vi "Channel by Index.vi"(8 "error in (no error)":errorcluster, 10 "Index":i32, 11 "StringGroup in":refnum<class "Group STR.lvclass">) -> (0 "error out":errorcluster, 2 "StringChannel":refnum<class "Channel STR.lvclass">, 3 "StringGroup out":refnum<class "Group STR.lvclass">)   [LabVIEW 2020, in "Vecto.lvlib" / "Group STR.lvclass"]
uses:
  Group STR.lvclass
  Channel STR/Channel STR.lvclass
  Channel STR/Channel STR.lvclass/Channel STR.ctl
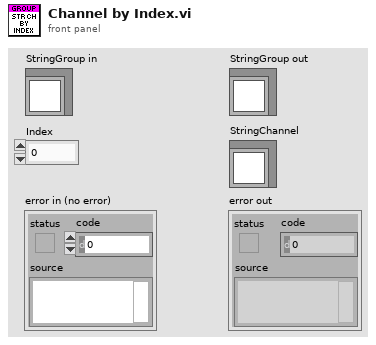
[diagram p1: front panel]
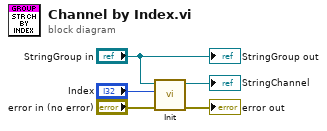
[diagram p0: block diagram]
diagram:
  n1 = call "Init.vi"("error in (no error)"="error in (no error)", "Index"="Index", "Group"="StringGroup in") -> ("error out"=→"error out":errorcluster, "StringChannel out"=→"StringChannel":refnum<class "Channel STR.lvclass">)  [unwired: 7 in]
  "StringGroup out" <- "StringGroup in"
